vi "电压结果判断.vi"(8 "判定阈值":u32[](array[numeric])=[320, 1, 1, 1], 9 "电压数组":u32[](array[numeric])) -> (2 "判定结果":bool, 3 "判定结果数组":bool[](array[boolean]))   [LabVIEW 2020]
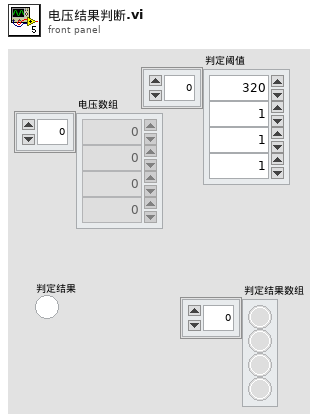
[diagram p1: front panel]
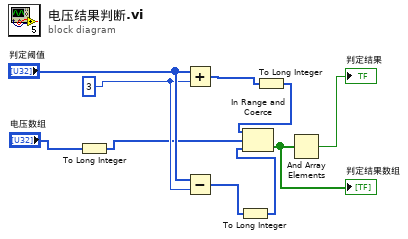
[diagram p0: block diagram]
diagram:
  w7 = 3
  n1 = To Long Integer(number="电压数组") -> (32bit integer=w1:i32[])
  n2 = Add(x="判定阈值", y=w7) -> (x+y=w4:u32[])
  n3 = Subtract(x="判定阈值", y=w7) -> (x-y=w6:u32[])
  n4 = To Long Integer(number=w6) -> (32bit integer=w5:i32[])
  n5 = To Long Integer(number=w4) -> (32bit integer=w3:i32[])
  n6 = In Range and Coerce(upper limit=w3, x=w1, lower limit=w5) -> (In Range?=w10:bool[])  [unwired: 1 out]
  "判定结果数组" <- w10
  n7 = And Array Elements(Boolean array=w10) -> (logical AND=→"判定结果":bool)
